vi "Call@SelectVI__Parameter.vi"(1 "ParamterIn":string) -> (0 "ParamterOut":string)   [LabVIEW 2019]
uses:
  MainFrame/Global.vi
panel:
  in  "Mode":string(combo)
  in  "VI":string(combo)
  in  "Confirm":bool
  # "Call@SelectVI $VI,$Parameter"
  # "Empty is Test Mode\n& is Normal Run\n&& is Call & Forget Mode"
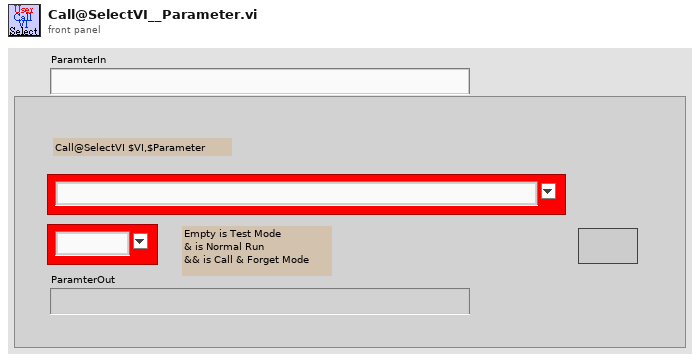
[diagram p1: front panel]
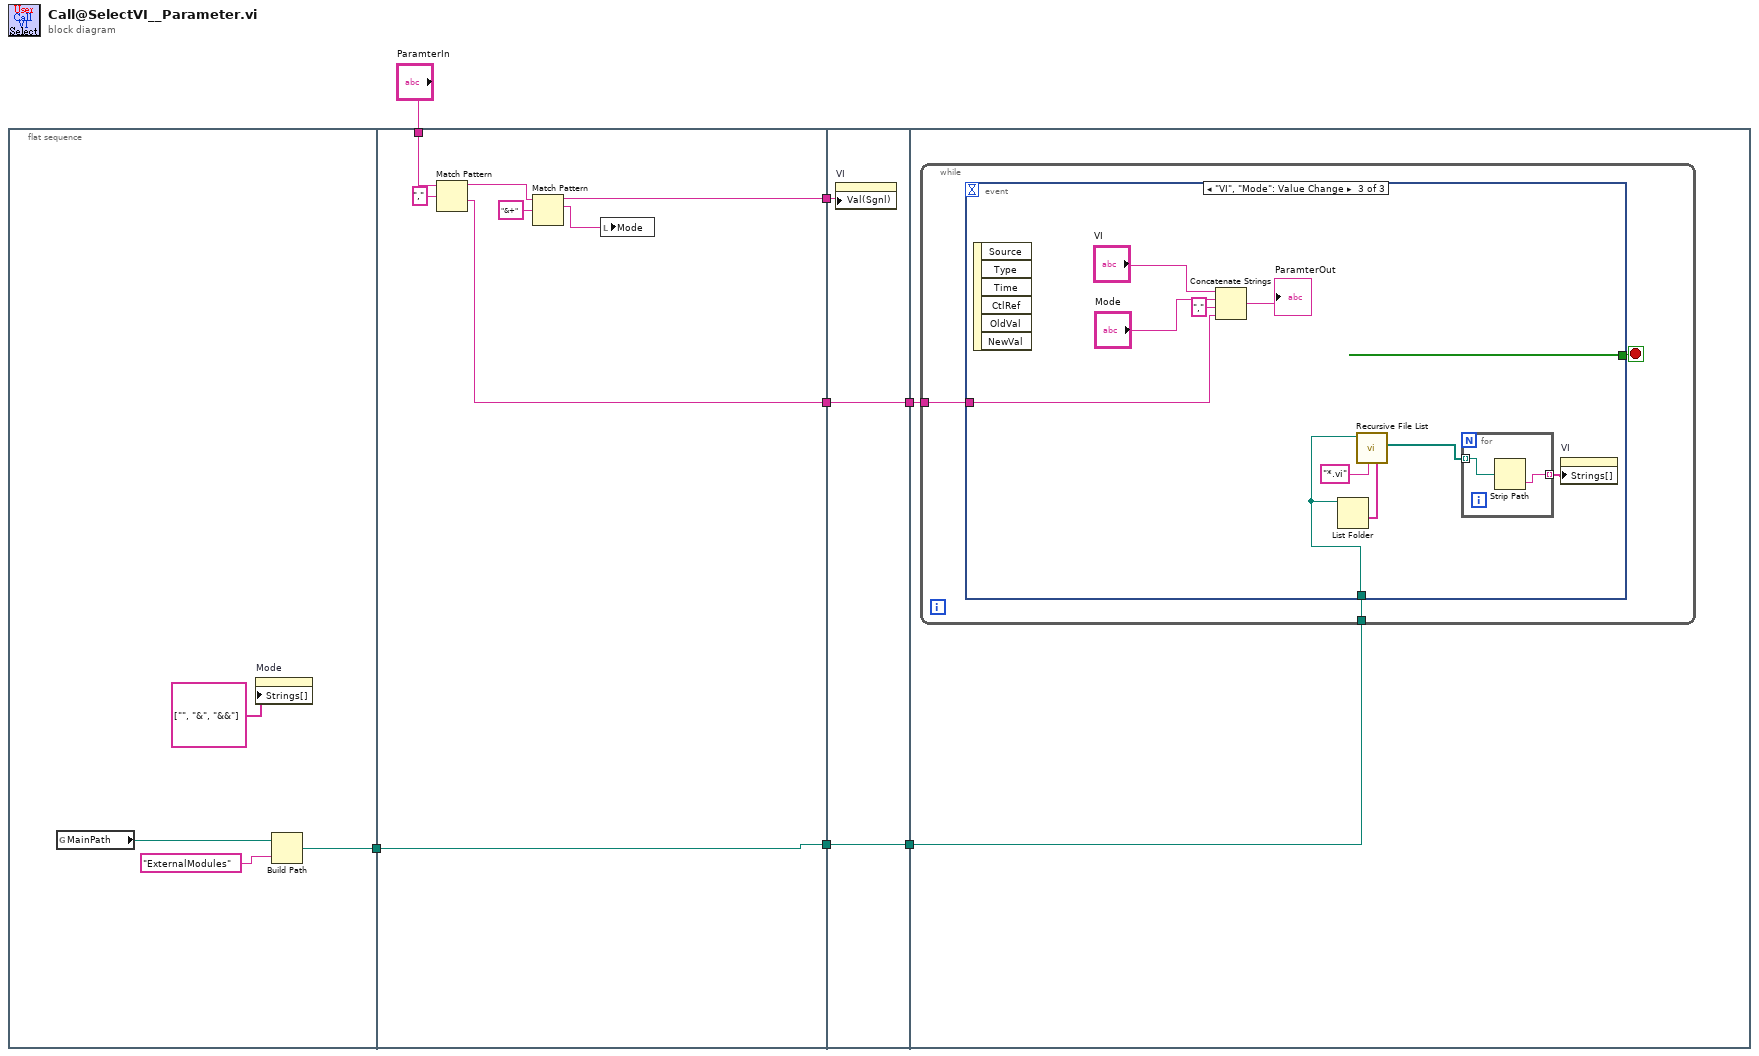
[diagram p0: block diagram]
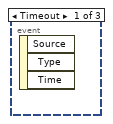
[diagram p2: hidden frame]
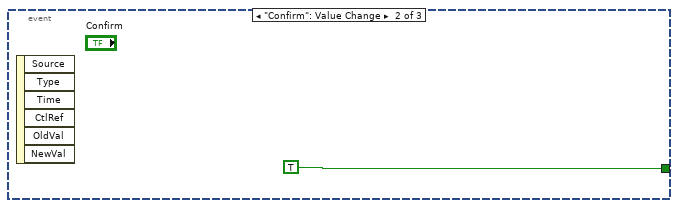
[diagram p3: hidden frame]
diagram:
  n1 = flat-sequence {
    tunnel: [w10] -> w4
    tunnel: "ParamterIn" -> [w18]
    tunnel: [w19] -> w5
    tunnel: w4 -> [w19]
    tunnel: [w16] -> w2
    tunnel: [w13] -> w1
    tunnel: [w22] -> w6
    tunnel: w5 -> [w22]
    tunnel: [w21] -> w3
    tunnel: w2 -> [w21]
    tunnel: w1 -> [w20]
    tunnel: w6 -> [w24]
    tunnel: w3 -> [w23]
    frame #0 {
      n2 = global read "Global.vi" "MainPath"() -> (w9:path)
      n3 = property on="Mode" class="CmbBox"("Strings[]"=string[] ["", "&", "&&"] ("Strings []")) -> ()  [unwired: 2 in, 2 out]
      n4 = Build Path(base path=w9, name or relative path="ExternalModules") -> (appended path=w10:path)
    }
    frame #1 {
      n5 = Match Pattern(string=w18, regular expression=",") -> (before substring=w15:string, after substring=w16:string)  [unwired: 1 in, 2 out]
      n6 = Match Pattern(string=w15, regular expression="&+") -> (before substring=w13:string, match substring=w12:string)  [unwired: 1 in, 2 out]
      n7 = local write "Mode"(w12) -> ()
    }
    frame #2 {
      n8 = property on="VI" class="CmbBox"("Val(Sgnl)"=w20) -> ()  [unwired: 2 in, 2 out]
    }
    frame #3 {
      n9 = while {
        tunnel: w24 -> [w26]
        tunnel: w23 -> [w25]
        stop <- w27 stop-if-true
        n10 = event shown="[2] \"VI\", \"Mode\": Value Change" {
          selector: _ -> [_ _ _]
          dyn-events: _ -> [_ _ _]
          timeout: _ -> [_ _ _]
          tunnel: [_ TRUE _] -> w27
          tunnel: w26 -> [_ _ w33]
          tunnel: w25 -> [_ _ w29]
          event Timeout {
            n11 = event-data() -> ()  [unwired: 1 in, 3 out]
          }
          event "Confirm": Value Change {
            n12 = event-data() -> ()  [unwired: 1 in, 6 out]
          }
          event "VI", "Mode": Value Change {
            n13 = event-data() -> ()  [unwired: 1 in, 6 out]
            n14 = Concatenate Strings("VI", "Mode", "," ("string"), w29) -> (→"ParamterOut":string)
            n15 = List Folder(path=w33) -> (folder names=w32:string[])  [unwired: 3 in, 3 out]
            n16 = call <vilib>:"Recursive File List.vi"("Folders to Exclude"=w32, "pattern"="*.vi", "Folder Path"=w33) -> ("All Files in Dir"=w36:path[])  [unwired: 4 in, 4 out]
            n17 = for {
              tunnel: w36 -> [w40] mode=indexing
              tunnel: [w39] -> w34 mode=indexing
              n18 = Strip Path(path=w40) -> (name=w39:string)  [unwired: 1 out]
            }
            n19 = property on="VI" class="CmbBox"("Strings[]"=w34) -> ()  [unwired: 2 in, 2 out]
          }
        }
      }
    }
  }
